vi "Write % Dead Zone Z-Axis.vi"(8 "error in (no error)":errorcluster, 10 "% Dead Zone Z-Axis":dbl, 11 "Joystick Guidance in":refnum<class "Joystick Guidance.lvclass">) -> (0 "error out":errorcluster, 3 "Joystick Guidance out":refnum<class "Joystick Guidance.lvclass">)   [LabVIEW 2011, in "Guidance Library.lvlib" / "Joystick Guidance.lvclass"]
uses:
  Joystick Guidance.lvclass
  Joystick Guidance.lvclass/Joystick Guidance.ctl
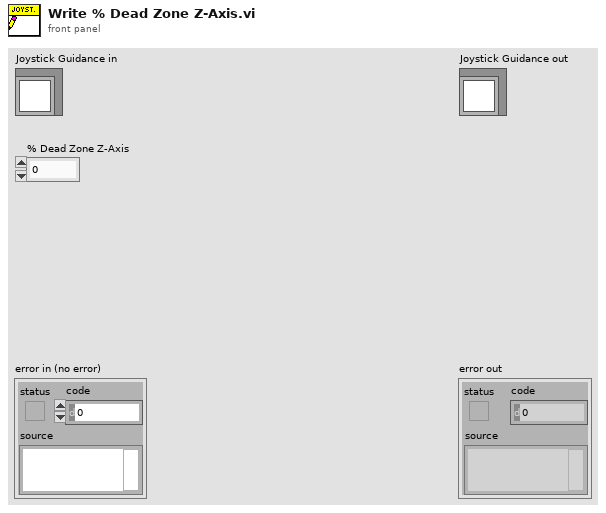
[diagram p1: front panel]
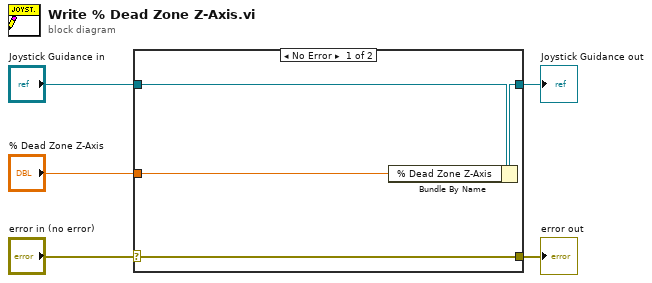
[diagram p0: block diagram]
diagram:
  n1 = case shown="No Error" "error in (no error)" {
    selector: "error in (no error)" -> [w9 w10]
    tunnel: [w9 w10] -> w4
    tunnel: [w7 w11] -> w2
    tunnel: "Joystick Guidance in" -> [w8 w11]
    tunnel: "% Dead Zone Z-Axis" -> [w6 _]
    frame No Error {
      n2 = Bundle By Name(cluster=w8, "% Dead Zone Z-Axis"=w6) -> (w7:refnum<class "Joystick Guidance.lvclass">)
    }
    frame Error {
    }
  }
  "error out" <- w4
  "Joystick Guidance out" <- w2
